vi "Write Teller Metadata In Msg.vi"(7 "Msg in":refnum<class "Msg.lvclass">, 10 "Teller Metadata":refnum<class "Teller Metadata.lvclass">) -> (5 "Msg out":refnum<class "Msg.lvclass">)   [LabVIEW 2020, in "jettl.lvlib"]
uses:
  jettl.lvlib
  Msg/Msg.lvclass
  Teller Metadata/Teller Metadata.lvclass
  Msg Input/Msg Input.lvclass
  Teller/Teller.lvclass
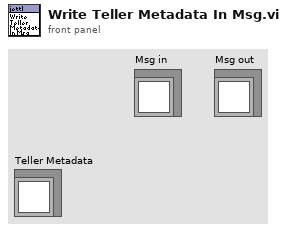
[diagram p1: front panel]
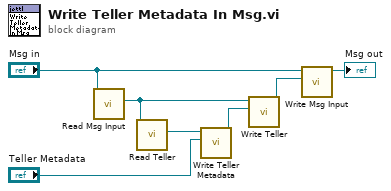
[diagram p0: block diagram]
diagram:
  n1 = call-dynamic "Read Msg Input.vi"("Msg in"="Msg in") -> ("Msg Input"=w4:refnum<class "Msg Input.lvclass">)  [unwired: 10 in]
  n2 = call-dynamic "Read Teller.vi"("Msg Input in"=w4) -> ("Teller"=w3:refnum<class "Teller.lvclass">)  [unwired: 10 in]
  n3 = call-dynamic "Write Teller Metadata.vi"("Teller Metadata"="Teller Metadata", "Teller in"=w3) -> ("Teller out"=w2:refnum<class "Teller.lvclass">)  [unwired: 9 in]
  n4 = call-dynamic "Write Teller.vi"("Teller"=w2, "Msg Input in"=w4) -> ("Msg Input out"=w5:refnum<class "Msg Input.lvclass">)  [unwired: 9 in]
  n5 = call-dynamic "Write Msg Input.vi"("Msg Input"=w5, "Msg in"="Msg in") -> ("Msg out"=→"Msg out":refnum<class "Msg.lvclass">)  [unwired: 9 in]
